vi "RES.vi"(7 "simulazione":bool, 8 "error in (no error)":errorcluster, 11 "Queue Name":string="RES_Q") -> (0 "error out":errorcluster)   [LabVIEW 2019]
uses:
  TypeDef/DEVICE NAME.ctl
  <vilib>/Utility/file.llb/Read Delimited Spreadsheet (string).vi
  Global_All_Data.vi
  Stop lettura res.vi
panel:
  out "Numeric":i32
  in  "Misura Resistomat":bool
  out "T max misura":i32
  out "Precisione mis":dbl
  out "N meas stab":i32
  out "T wait start (s)":i32
  in  "Mode sing?":bool
  out "Reset Device (Don't Reset)":bool
  out "Group Address (0)":i32
  out "Time-out (1.0)":dbl
  out "Baud Rate (9600)":i32
  out "n meas":string
  out "errore resistomat":bool
  out "SCALA":u16
  out "COM-Port (0)":i32
  out "Iteration":i32
  in  "RANGE":u16(ring) items=["20 mOhm", "200 mOhm", "2 Ohm", "20 Ohm", "200 Ohm", "2 kOhm", "20 kOhm", "200 kOhm"]
  in  "CONFIGURE":bool
  in  "stop":bool
  in  "MEASURE":bool
  out "Measuring Value":dbl format="%#_6f OHM"
  out "Communication settings":T1={"COM-Port (0)"=0, "Baud Rate (9600)"=9600, "Time-out (1.0)"=1.0, "Group Address (0)"=0, "Reset Device (Don't Reset)"=FALSE} {"Baud Rate (9600)" items=["1200"=1200, "2400"=2400, "4800"=4800, "9600"=9600, "19200"=19200, "38400"=38400, "56000"=56000, "57600"=57600]; "COM-Port (0)" min=1 max=32 step=1}
  out "N° in queue":i32
  out "variant":variant
  out "STATO":string
  out "LOOP TIME (ms)":u32
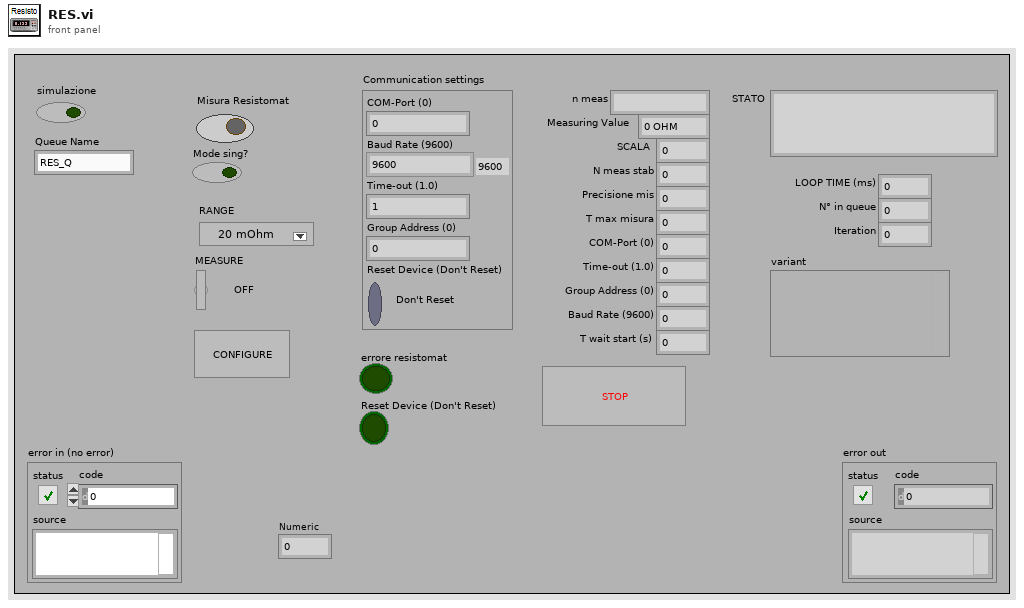
[diagram p1: front panel]
types:
  T1 = cluster{"COM-Port (0)":i32, "Baud Rate (9600)":i32, "Time-out (1.0)":dbl, "Group Address (0)":i32, "Reset Device (Don't Reset)":bool}
  T2 = typedef "DEVICE NAME.ctl" = enum16{"WATTMETRO", "APLUS", "PLC BANCO 1", "PLC RACK", "PLC BANCO 2", "PS", "NI cDAQ", "RESISTOMAT"}
  T3 = typedef "Cluster MISURE.ctl" = cluster{"MISURE NM":T4, "MISURE ALL":T5}
  T4 = typedef "MISURE NM.ctl" = cluster{"Banco":string, "Anno":string, "Numero":string, "Ntabella":string, "Misura":string, "Tipo Prova":string, "ProgressivoAcq":string, "Descrizione":string, "Data_ora":string, "t. acq [h:m:s]":string, "t. acq [min]":string, "t. acq [s]":string, "n [rpm]":string, "f [Hz]":string, "U1[V]":string, "U2 [V]":string, "U3 [V]":string, "U123_media [V]":string, "I1[A]":string, "I2[A]":string, "I3[A]":string, "I123_media [A]*I":string, "I_123_sbil [%]":string, "Ulin[V]":string, "Uc [V]":string, "Uaux [V]":string, "Ilin[A]*I":string, "Imar[A]":string, "Iaux[A]":string, "Uarm[V]":string, "Uecc[V]":string, "Iarm[A]*I":string, "Iecc[A]":string, "pf":string, "P1 [W]":string, "P1 [kW]":string, "Q [VAR]":string, "Q [kVAR]":string, "S [VA]":string, "S [kVA]":string, "P1arm[W]":string, "P1ecc[W]":string, "Parm[kW]":string, "P1ecc[kW]":string, "Cond[uF]":string, "P1_linea_6fili[W]":string, "P1_linea_6fili[kW]":string, "eta_gr_6fili [%]":string, "eta_inverter_6fili [%]":string, "pf_linea_6fili":string, "U4 [V]":string, "U5 [V]":string, "U6 [V]":string, "U456_media [V]":string, "I4 [A]":string, "I5 [A]":string, "I6 [A]":string, "I456_media [A]":string, "C [Nm]*C":string, "Cric [Nm]":string, "Cric\\Cnom":string, "Iric[A]":string, "Iric\\Inom":string, "P2_mecc [W]":string, "P2_mecc [kW]":string, "eta motore [%]":string, "Scorr[%]":string, "Tamb[°C]":string, "R1[ohm]":string, "R2[ohm]":string, "R3[ohm]":string, "Rmedia[ohm]":string, "DT_R1[°C]":string, "DT_R2[°C]":string, "DT_R3[°C]":string, "DT_media[°C]":string, "R_marcia[ohm]":string, "R_aux[ohm]":string, "DT_marcia[°C]":string, "DT_aux[°C]":string, "R_Arm[ohm]":string, "R_Ecc[ohm]":string, "DT_Arm[°C]":string, "DT_Ecc[°C]":string, "TambFreddo[°C]":string, "R1_freddo[ohm]":string, "R2_freddo[ohm]":string, "R3_freddo[ohm]":string, "Rmedia_freddo[ohm]":string, "R_Marcia_freddo[ohm]":string, "R_Aux_freddo[ohm]":string, "R_Arm_freddo[ohm]":string, "R_Ecc_freddo[ohm]":string, "TC1 [°C]":string, "TC2 [°C]":string, "TC3 [°C]":string, "TC4 [°C]":string, "TC5 [°C]":string, "TC6 [°C]":string, "TC7 [°C]":string, "TC8 [°C]":string, "PT1000_1[°C]":string, "PT1000_2[°C]":string, "PT1000_3[°C]":string, "Vdc eccitatrice[V]":string, "Idc eccitatrice[A]":string, "Vdc rotore[V]":string, "Idc rotore[A]":string, "Vac rotore[V]":string, "Iac rotore[V]":string, "V dinamo[V]":string, "Portata Q":string, "Pressione H":string, "U1'[V]":string, "U2'[V]":string, "U3'[V]":string, "I1'[A]":string, "I2'[A]":string, "I3'[A]":string, "U''R-N":string, "U''S-N":string, "U'' T-N":string, "U''R-S":string, "U''R-T":string, "U''S-T":string, "I1''[A]":string, "I2''[A]":string, "I3''[A]":string, "F''[Hz]":string, "P''[kW]":string, "CosFi''":string, "PT1000_4[°C]":string, "Scorta 3":string}
  T5 = typedef "Cluster misure ALL.ctl" = cluster{"Cluster READ NI":T6, "MISURE WT":T9, "Resistenze Resistomat":T10, "INTERFACCIA":T11, "FREDDO resistomat":cluster{"Res Ch1":dbl, "Res Ch2":dbl, "tAMB":dbl, "Res Ch3":dbl}, "STATO PLC 1":T16, "Res Ch2":dbl, "Res Ch2 2":dbl, "FREDDO res meter":cluster{"Res Ch1":dbl, "Res Ch2":dbl, "tAMB":dbl, "Res Ch3":dbl}, "Resistenze Res Meter":T10, "READ SINUS PENTA":T20, "STATO PLC 2":T21, "STATO PLC 3":T25, "DCREG":T29}
  T6 = typedef "Cluster NI.ctl" = cluster{"AI (0-10V)":cluster{"AI 0":dbl, "AI 1":dbl, "AI 2":dbl, "AI 3":dbl, "AI 4":dbl, "AI 5":dbl, "AI 6":dbl, "AI 7":dbl, "AI 8":dbl, "AI 9":dbl, "AI 10":dbl, "AI 11":dbl, "AI 12":dbl, "AI 13":dbl, "AI 14":dbl, "AI 15":dbl, "AI 16":dbl, "AI 17":dbl, "AI 18":dbl, "AI 19":dbl, "AI 20":dbl, "AI 21":dbl, "AI 22":dbl, "AI 23":dbl, "AI 24":dbl, "AI 25":dbl, "AI 26":dbl, "AI 27":dbl, "AI 28":dbl, "AI 29":dbl, "AI 30":dbl, "AI 31":dbl}, "StatoAO_Cdaq[0-10V]":cluster{"AO 1":dbl, "AO 2":dbl, "AO 3":dbl, "AO 4":dbl}, "Contatori [rpm]":cluster{"RPM 1":dbl, "RPM 2":dbl}, "StatoAO_Cdaq [4-20mA]":T7, "StatoDO_Cdaq":T8, "DI":cluster{"Scorta 0":bool, "Scorta 1":bool, "Scorta 2":bool, "Scorta 3":bool, "Scorta 4":bool, "Scorta 5":bool, "Scorta 6":bool, "Scorta 7":bool, "Scorta 8":bool, "Scorta 9":bool, "Scorta 10":bool, "Scorta 11":bool, "Scorta 12":bool, "Scorta 13":bool, "Scorta 14":bool, "Scorta 15":bool, "Scorta 16":bool, "Scorta 17":bool, "Scorta 18":bool, "Scorta 19":bool, "Scorta 20":bool, "Scorta 21":bool, "Scorta 22":bool, "Scorta 23":bool, "Scorta 24":bool, "Scorta 25":bool, "Scorta 26":bool, "Scorta 27":bool, "Scorta 28":bool, "Scorta 29":bool, "Scorta 30":bool, "Scorta 31":bool}, "AI (4-20mA)":cluster{"AI 0":dbl, "AI 1":dbl, "AI 2":dbl, "AI 3":dbl, "AI 4":dbl, "AI 5":dbl, "AI 6":dbl, "AI 7":dbl, "AI 8":dbl, "AI 9":dbl, "AI 10":dbl, "AI 11":dbl, "AI 12":dbl, "AI 13":dbl, "AI 14":dbl, "AI 15":dbl}, "TC [°C]":cluster{"tc 1":dbl, "tc 2":dbl, "tc 3":dbl, "tc 4":dbl}, "NI Read Values":cluster{"RPM":dbl, "Frequency":dbl, "Mod 1":cluster{"Torsiometro 1":dbl, "Torsiometro 2":dbl, "Strin Gauge 1":dbl, "Strin Gauge 2":dbl}, "Mod 2":cluster{"Termocoppia 1":dbl, "Termocoppia 2":dbl, "Termocoppia 3":dbl, "Termocoppia 4":dbl}, "Mod 3":cluster{"PT 100 1":dbl, "PT 100 2":dbl, "PT 100 3":dbl, "PT 100 4":dbl}}}
  T7 = typedef "StatoAO_cdaq.ctl" = cluster{"Cdaq_AO [0-10V] 0 for Torque":dbl, "Cdaq_AO [0-10V] 1":dbl, "Cdaq_AO [0-10V] 2":dbl, "Cdaq_AO [0-10V] 3":dbl}
  T8 = typedef "statoDO_Cdaq.ctl" = cluster{"Scorta 0":bool, "Scorta 1":bool, "Scorta 2":bool, "Scorta 3":bool, "Scorta 4":bool, "Scorta 5":bool, "Scorta 6":bool, "Scorta 7":bool, "Scorta 8":bool, "Scorta 9":bool, "Scorta 10":bool, "Scorta 11":bool, "Scorta 12":bool, "Scorta 13":bool, "Scorta 14":bool, "Scorta 15":bool, "Scorta 16":bool, "Scorta 17":bool, "Scorta 18":bool, "Scorta 19":bool, "Scorta 20":bool, "Scorta 21":bool, "Scorta 22":bool, "Scorta 23":bool, "Scorta 24":bool, "Scorta 25":bool, "Scorta 26":bool, "Scorta 27":bool, "Scorta 28":bool, "Scorta 29":bool, "Scorta 30":bool, "Scorta 31":bool}
  T9 = typedef "MISURE WT.ctl" = cluster{"URMS 1":dbl, "IRMS 1":dbl, "P 1":dbl, "S 1":dbl, "Q 1":dbl, "LAMBDA 1":dbl, "PHI 1":dbl, "F U 1":dbl, "F I 1":dbl, "NONE 1":dbl, "URMS 2":dbl, "IRMS 2":dbl, "P 2":dbl, "S 2":dbl, "Q 2":dbl, "LAMBDA 2":dbl, "PHI 2":dbl, "F U 2":dbl, "F I 2":dbl, "NONE 2":dbl, "URMS 3":dbl, "IRMS 3":dbl, "P 3":dbl, "S 3":dbl, "Q 3":dbl, "LAMBDA 3":dbl, "PHI 3":dbl, "F U 3":dbl, "F I 3":dbl, "NONE 3":dbl, "URMS SIGMA":dbl, "IRMS SIGMA":dbl, "P SIGMA":dbl, "S SIGMA":dbl, "Q SIGMA":dbl, "LAMBDA SIGMA":dbl, "PHI SIGMA":dbl, "F U SIGMA":dbl, "F I SIGMA":dbl, "NONE 4":dbl}
  T10 = typedef "ClusterRes.ctl" = cluster{"Res Ch1":dbl, "Res Ch2":dbl, "Res Ch3":dbl, "Tamb":dbl}
  T11 = typedef "INTERFACCIA.ctl" = cluster{"AI":cluster{"Portate":T12[], "Pressioni":T12[], "Coppie[Nm]":T12[], "Valvole prop %":T12[], "RPM":T12[], "Livelli":T12[], "Temperature":T12[], "Riferimenti %":T12[], "TENSIONI":T12[], "CORRENTI":T12[]}, "DI (logici)":cluster{"Start da pulsantiera":bool, "Stop da pulsantiera":bool, "Reset da pulsantiera":bool, "Sistema OK":bool, "Collaudo abilitato":bool, "Potenza trifase abilitata":bool, "Potenza monofase abilitata":bool, "Potenza DC abilitata":bool, "Potenza DC ECC abilitata":bool, "Start alimentazione AC":bool, "Start alimentazione DC":bool, "Start DC eccitazione":bool, "Teleruttore WT abilitato":bool, "Teleruttore Resistomat abilitato":bool, "Teleruttore corto fasi":bool, "Ramo 1 resistomat":bool, "Ramo 2 resistomat":bool, "Ramo 3 resistomat":bool, "B1 Scelta linea elettrica 1":bool, "B1 Scelta linea elettrica 2":bool, "B1 Scelta linea elettrica 3":bool, "B1 Scelta linea elettrica 4":bool, "B1 Scelta linea elettrica 5":bool, "B2 Scelta linea elettrica 1":bool, "B2 Scelta linea elettrica 2":bool, "B2 Scelta linea elettrica 3":bool, "B2 Scelta linea elettrica 4":bool, "B2 Scelta linea elettrica 5":bool, "Rotore bloccato 1":bool, "Rotore bloccato 2":bool, "FRENO 1 abilitato":bool, "FRENO 1 run":bool, "FRENO 1 senso rotaz":bool, "FRENO 1 ctrl velocità":bool, "FRENO 2 abilitato":bool, "FRENO 2 run":bool, "FRENO 2 senso rotaz":bool, "FRENO 2 ctrl velocità":bool, "ALIM 1 abilitato":bool, "ALIM 1 run":bool, "ALIM 2 abilitato":bool, "ALIM 2 run":bool, "ALIM 3 abilitato":bool, "ALIM 3 run":bool, "FRENO 1 ctrl coppia":bool, "FRENO 2 ctrl coppia":bool, "FRENO 3 ctrl coppia":bool, "DI (logici) aggiuntivi impianto":cluster{"Solo freno abilitato":bool, "Carico resistivo abilitato":bool, "AFE+freno abilitato":bool, "Protezioni chiuse":bool, "Start potenza AFE":bool, "AFE in marcia":bool}, "Misura corrente diretta WT":bool, "Misura corrente sens ext":bool, "Sens ext abilitati":bool}, "AO non scalati":T14, "AO scalati":T14, "DO (logici)":T15}
  T12 = typedef "ClusterMisura_e_Unità_INPUT.ctl" = cluster{"Misura":dbl, "UM":T13, "Descrizione":string}
  T13 = typedef "UnitàMisura.ctl" = enum16{"V", "mA", "Bar", "RPM", "m3/s", "m3/min", "m3/h", "l/s", "l/min", "in3/min", "ft3/min", "gpm", "igpm", "igph", "%", "°C", "m", "Nm", "A"}
  T14 = typedef "Lista AO sistema.ctl" = cluster{"FRENO1 rif vel":dbl, "FRENO1 rif Coppia":dbl, "FRENO2 rif vel":dbl, "FRENO2 rif Coppia":dbl, "ALIM1 rif V":dbl, "ALIM1 rif F":dbl, "ALIM2 rif V":dbl, "ALIM2 rif F":dbl, "ALIM3 rif V":dbl, "ALIM3 rif F":dbl, "Fnom keb":dbl, "Rpm nom keb":dbl, "Pnom keb":dbl, "Inom keb":dbl, "Vnom keb":dbl, "Rpm max keb":dbl, "Tempo rampa keb":dbl, "Tipo Mot keb":dbl, "FRENO  rif Coppia ":dbl, "FRENO  rif  Corrente":dbl}
  T15 = typedef "DOinterfaccia.ctl" = cluster{"Scelta banco 1":bool, "Scelta banco 2":bool, "Scelta banco 3":bool, "FRENO 1 abilita":bool, "FRENO 1 start":bool, "FRENO 1 senso rotaz":bool, "FRENO 1 ctrl velocità":bool, "FRENO 2 abilita":bool, "FRENO 2 start":bool, "FRENO 2 senso rotaz":bool, "FRENO 2 ctrl velocità":bool, "ALIM 1 abilita":bool, "ALIM 1 start":bool, "ALIM 2 abilita":bool, "ALIM 2 start":bool, "ALIM 3 abilita":bool, "ALIM 3 start":bool, "Abilita linea trifase":bool, "Abilita linea monofase":bool, "Abilita linea dc":bool, "Abilita linea dc eccit":bool, "B1 Linea elettrica 1":bool, "B1 Linea elettrica 2":bool, "B1 Linea elettrica 3":bool, "B1 Linea elettrica 4":bool, "B1 Linea elettrica 5":bool, "B2 Linea elettrica 1":bool, "B2 Linea elettrica 2":bool, "B2 Linea elettrica 3":bool, "B2 Linea elettrica 4":bool, "B2 Linea elettrica 5":bool, "Start potenza AC":bool, "Stop pontenza AC":bool, "Start potenza DC":bool, "Stop potenza DC":bool, "Start potenza eccitaz":bool, "Stop potenza eccitaz":bool, "Reset allarmi":bool, "watchdog":bool, "Scala torsiometro B1":bool, "Controllo torsiom B1":bool, "Scala torsiometro B2":bool, "Controllo torsiom B2":bool, "Teleruttore WT abilita":bool, "Teleruttore Resistomat abilita":bool, "Teleruttore corto fasi":bool, "Ramo 1 resistomat":bool, "Ramo 2 resistomat":bool, "Ramo 3 resistomat":bool, "Collaudo in corso":bool, "Allarme presente":bool, "Enable Res Meter":bool, "Bypass Res Meter":bool, "2nd canale Res Meter":bool, "Scala 200/2000 res meter":bool, "Taratura res meter":bool, "FRENO 1 ctrl coppia":bool, "FRENO 2 ctrl coppia":bool, "FRENO 3 ctrl coppia":bool, "Aggiuntivi impianto":cluster{"Senso rotazione alim 1":bool, "Senso rotazione alim 2":bool}, "ALIM 1 stop":bool, "ALIM 2 stop":bool, "ALIM 3 stop":bool, "FRENO 1 stop":bool, "FRENO 2 stop":bool, "FRENO 3 stop":bool, "B1 configurazione freno B":bool, "B2 configurazione freno B":bool, "Abilita scrittura KEB":bool, "Bench Selection (0-B1,1-B2)":bool, "Select current mode":bool, "Select torque mode":bool, "Select speed mode":bool, "Start":bool, "Stop":bool, "Block":bool, "Enable Force mode":bool, "Abilita linea 125 A":bool, "Abilita linea 63 A":bool, "Abilita linea 16 A":bool, "Aum Tensione Variac":bool, "Dim Tesnione Variac":bool, "Abilita ellectro stractura":bool, "Risprinito Emergence":bool, "Abilita collaudo":bool, "Disabilita collaudo":bool, "External Alaram":bool, "Enable external program":bool, "Reset":bool, "Abilita Ingresso Variac":bool, "Abilita Ventilatore Variac":bool, "Abilita Uscita Variac ":bool}
  T16 = typedef "STATO PLC 1.ctl" = cluster{"USCITE PLC":T17, "Stato DI_PLC":cluster{"Sistema OK":bool, "Rotore bloccato":bool, "Scorta 1":bool, "Prova diretto inverter":bool, "Prova con filtro LC":bool, "Teleruttore WT abilitato":bool, "Alim sinus penta abilitato":bool, "Alim sinus penta in marcia":bool, "Freno abilitato":bool, "Freno in marcia":bool, "Senso rotazione freno":bool, "Potenza abilitata":bool, "Scorta 3":bool, "Scorta 4":bool, "scorta 5":bool, "scorta 6":bool}, "AI plc":cluster{"Allarmi 1":dbl, "Allarmi 2":dbl, "Scorta 1":dbl, "Scorta 2":dbl, "RPM mot prova":dbl, "I mot prova":dbl, "RPM freno":dbl, "I freno":dbl, "Scorta 3":dbl, "Scorta 4":dbl}}
  T17 = typedef "Uscite PLC 1.ctl" = cluster{"AO (real) 2":cluster{"SCORTA 1":dbl, "SCORTA 2":dbl, "SCORTA 3":dbl, "SCORTA 4":dbl, "SCORTA 5":dbl, "SCORTA 6":dbl, "SCORTA 7":dbl, "SCORTA 8":dbl}, "statoAO_PLC out":T18, "DO (bit)":T19}
  T18 = typedef "statoAO_plc_1.ctl" = cluster{"Rif Lim coppia freno [%]":dbl, "Rif rpm freno [%]":dbl, "Rif coppia freno [%]":dbl, "Rif V alimentatore [%]":dbl, "Rif F alimentatore [%]":dbl}
  T19 = typedef "StatoDO_PLC_1.ctl" = cluster{"Scelta banco 1":bool, "Set dati motore freno 2":bool, "Diretto inverter":bool, "Filtro LC":bool, "Marcia ALIM (1s)":bool, "Marcia FRENO (1s)":bool, "Stop AFE (1s)":bool, "Stop freno (1s)":bool, "Reset allarmi":bool, "Watchdog":bool, "Senso rotazione":bool, "Abilita collaudo (1s)":bool, "Disabilita collaudo (1s)":bool, "Abilitazione ALIM":bool, "Abilitazione FRENO":bool, "Teleruttore WT":bool, "Senso rot motore prova":bool, "Scorta 7":bool, "Scorta 8":bool, "Scorta 9":bool, "Scorta 10":bool, "Scorta 11":bool, "Scorta 12":bool, "Scorta 13":bool}
  T20 = typedef "Parametri inverter letti.ctl" = cluster{"Menù Misure motore (M000-M030)":cluster{"Rif vel a regime (int)":u16, "Rif vel a regime (dec)":u16, "Rif vel dopo rampe (int)":u16, "Rif vel dopo rampe (dec)":u16, "RPM motore (int)":u16, "RPM motore (dec)":u16, "FREQout inverter":u16, "Rif coppia a regime(Nm)":u16, "Richiesta di coppia (Nm)":u16, "Coppia generata dal motore(Nm)":u16, "Rif coppia a regime(%)":u16, "Richiesta di coppia (%)":u16, "Coppia generata dal motore(%)":u16, "Coppia max richiesta prima delle rampe(Nm)":u16, "Coppia max richiesta dopo le rampe(Nm)":u16, "Limite di velocità prima delle rampe":u16, "Limite di velocità dopo le rampe":u16, "Coppia max richiesta prima delle rampe(%)":u16, "Coppia max richiesta dopo le rampe(%)":u16, "Rif di flusso":u16, "Corrente di uscita":u16, "Capacità termica del motore":u16, "Tensione di uscita":u16, "Potenza di uscita":u16, "Energia consumata (LSword)":u16, "Energia consumata (MSword)":u16, "Tensione bus DC":u16, "Tensione di rete":u16}, "Menù regolatore PID (M018-M024)":cluster{"Rif PID a regime(%)":u16, "Rif pid dopo rampe(%)":u16, "Retroazione del pid(%)":u16, "Errore del pid(%)":u16, "uscita del pid(%)":u16, "Rif del pid dopo le rampe":u16, "Retroazione del pid":u16}, "Menù ingressi digitali (M031-M036)":cluster{"Ingressi digitali ritardati":u16, "Ingressi digitali istantanei":u16, "Moresettiera comando loc":u16, "Morsett comando da seriale":u16, "Morsett comando bus di campo":u16, "Ing dig ausiliari da morsettiera":u16, "Ing dig ausiliari da seriale":u16}, "Menù riferimenti (M037-M051)":cluster{"Rif analog est REF":u16, "Rif analog est AIN1":u16, "Rif analog est AIN2":u16, "Rif analog est XAIN4":u16, "Rif analog est XAIN5":u16, "Rif velocità da seriale(int)":u16, "Rif velocità bus di campo(int)":u16, "Rif coppia da seriale":u16, "Rif coppia bus di campo":u16, "Rif del PID da seriale":u16, "Rif del PID da bus di campo":u16, "Retroazione del PID da seriale":u16, "Retroazione del PIDda bus di campo":u16, "Rif da encoder":u16, "Rif in frequenza":u16, "Rif velocità da seriale(dec)":u16, "Rif velocità bus di campo(dec)":u16}, "Menù rampe (P009-P033)":cluster{"Tempo di dec rampa di vel 1":u16, "Tempo di acc rampa di vel 2":u16, "Tempo di dec rampa di vel 2":u16, "Tempo di acc rampa di vel 1":u16, "Unità di mis tempi rampe vel 1/2":u16, "Tempo di acc rampa di vel 3":u16, "Tempo di dec rampa di vel 3":u16, "Tempo di acc rampa di vel 4":u16, "Tempo di dec rampa di vel 4":u16, "Unità di mis tempi rampe vel 3/4":u16, "Selettore arrottondam rampe":u16, "Tempo di arrotond iniz rampa acc":u16, "Tempo di arrotond finale rampa acc":u16, "Tempo di arrotond iniz rampa dec":u16, "Tempo di rampa di salita rif coppia":u16, "Tempo di rampa di discesa rif coppia":u16, "Unità di misura rampa coppia":u16, "Tempo rampa acc marcia jog":u16, "Tempo rampa dec marcia jog":u16, "Reset acc ai cambi pendenza":u16, "rampa di acc in fire mode":u16, "rampa di dec in fire mode":u16, "Tempo di arrotond finale rampa dec":u16}, "Menù controllo motore(C008-C128)":cluster{"Numero motori configurati":u16, "Tipo algoritmo di controllo Mot1":u16, "Tipo rif Mot1":u16, "Tensione nominale rete":u16, "Retroaz di vel da encoder Mot1":u16, "Tipo curva V/f Mot1":u16, "Rotazione delle fasi Mot1":u16, "Freq nominale del motore Mot1":u16, "RPM nominali del motore Mot1":u16, "Potenza nominale del motore Mot1":u16, "Corrente nominale del motore Mot1":u16, "Tensione nominale del motore mot1":u16, "Potenza a vuoto del motore Mot1":u16, "Corrente a vuoto del motore Mot1":u16, "Resistenza statorica del motore Mot1":u16, "Induttanza di dispersione Mot1":u16, "Induttanza mutua motore":u16, "Costante di tempo rotorica":u16, "Costante di tempo filtro pb":u16, "Velocità minima motore":u16, "Velocità massima motore":u16}, "Menù configurazione PID":cluster{"Selezione riferimento n.1":u16, "Selezione retroazione n.1":u16, "Modalità di fuzionamento PID":u16, "Termine derivativo calcolato su err o mis":u16, "Proporz moltiplica deriv e integrale":u16, "Azione del PID":u16}, "ID":dbl, "Menù uscite digitali":cluster{"MDO4 Inverter pronto":u16}, "Fcarrier":cluster{"Fcarrier Min (Hz)":u16, "Fcarrier Max (Hz)":u16}, "stato inverter M089":dbl, "Riferimenti":cluster{"Rif tensione":u16, "Rif velocità":u16}, "Comunicazione":bool, "Modalità stop":dbl}
  T21 = typedef "STATO PLC 2.ctl" = cluster{"USCITE PLC":T22, "Stato DI_PLC":cluster{"Sistema ok":bool, "Relè Resistomat abilitato":bool, "Freno abilitato":bool, "Freno in marcia":bool, "scorta b":bool, "scorta a":bool, "scorta 1":bool, "scorta 2":bool, "scorta 3":bool, "scorta 4":bool, "Scorta 5":bool, "Scorta 6":bool, "Scorta 7":bool, "Scorta 8":bool, "Scorta 9":bool, "Scorta 10":bool}, "AI plc":cluster{"Allarmi 1":dbl, "Allarmi 2":dbl, "TC 1":dbl, "TC 2":dbl, "TC 3":dbl, "TC 4":dbl, "TC 5":dbl, "TC 6":dbl, "TC 7":dbl, "TC 8":dbl, "PT1000 1":dbl, "PT1000 2":dbl, "PT1000 3":dbl, "PT1000 4":dbl}}
  T22 = typedef "Uscite PLC 2.ctl" = cluster{"AO (real) 2":cluster{"SCORTA 1":dbl, "SCORTA 2":dbl, "SCORTA 3":dbl, "SCORTA 4":dbl, "SCORTA 5":dbl, "SCORTA 6":dbl, "SCORTA 7":dbl, "SCORTA 8":dbl}, "statoAO_PLC out":T23, "DO (bit)":T24}
  T23 = typedef "statoAO_plc_2.ctl" = cluster{"Condensatori":dbl, "Scorta 1":dbl, "Scorta 2":dbl}
  T24 = typedef "StatoDO_PLC_2.ctl" = cluster{"Relè misura resistomat":bool, "Misura res ramo 1":bool, "Misura res ramo 2":bool, "Misura res ramo 3":bool, "Scelta banco 2":bool, "Scala Torsiometro":bool, "Ctrl torsiometro":bool, "Select current mode":bool, "Select Torque mode":bool, "Select speed mode":bool, "Watchdog":bool, "Scorta":bool, "Scorta 2":bool, "Scorta 3":bool, "Scorta 4":bool, "Scorta 5":bool, "Bench selection":bool, "External alarm":bool, "Enable external program":bool, "Reset allarmi":bool, "Start":bool, "Stop":bool, "Block":bool, "Scorta 6":bool}
  T25 = typedef "STATO PLC 3.ctl" = cluster{"USCITE PLC":T26, "Stato DI_PLC":cluster{"Sistema OK":bool, "Rotore bloccato":bool, "Filtro LC":bool, "Bypass Filtro LC":bool, "Scelta Trasformatore":bool, "Scelta Bypass trasformatore":bool, "Teleruttore wt abilitato":bool, "Alimentatore abilitato":bool, "Alimentatore in marcia":bool, "Scorta 1":bool, "Scorta 2":bool, "Scorta 3":bool, "Potenza abilitata":bool, "Alimentatore in allarme":bool, "Scorta 4":bool, "Conferma dati KEB":bool, "Scorta 5":bool, "Warning Inverter Alimentatore":bool, "Variac Abilitato":bool, "Linea 125 A abilitata":bool, "Linea 63 A abilitata":bool, "Linea 16 A abilitata":bool, "Scorta 6":bool, "Enable force mode":bool}, "AI plc":cluster{"Allarmi 1":dbl, "Allarmi 2":dbl, "RPM motore prova":dbl, "Corrente motore prova":dbl, "RPM freno":dbl, "Corrente freno":dbl, "Tipo motore keb":dbl, "I nom keb":dbl, "RPM nom keb":dbl, "V nom keb":dbl, "F nom keb":dbl, "T rampa keb":dbl, "scorta":dbl, "Scorta 2":dbl}}
  T26 = typedef "Uscite PLC 3.ctl" = cluster{"AO (real) 2":cluster{"SCORTA 1":dbl, "SCORTA 2":dbl, "SCORTA 3":dbl, "SCORTA 4":dbl, "SCORTA 5":dbl, "SCORTA 6":dbl, "SCORTA 7":dbl, "SCORTA 8":dbl}, "statoAO_PLC out":T27, "DO (bit)":T28}
  T27 = typedef "statoAO_plc_3.ctl" = cluster{"Rif velocità alimentatore":dbl, "Scorta":dbl, "Tipo Motore  keb":dbl, "I nom keb":dbl, "RPM nom keb":dbl, "V nom keb":dbl, "F nom keb":dbl, "t rampa keb":dbl}
  T28 = typedef "StatoDO_PLC_3.ctl" = cluster{"Select linea Inverter":bool, "Abilita sense wattmetro":bool, "Bypass filtro LC":bool, "Filtro LC":bool, "Bypass trasformatore":bool, "Trasformatore":bool, "Abilita uscite variac":bool, "Abilita linea 125 A":bool, "Abilita linea 63 A":bool, "Abilita linea 16 A":bool, "Abilita Scrittura Dati Keb":bool, "Abilita alimentatore":bool, "Marcia alimentatore (1s)":bool, "Stop alimentatore (1s)":bool, "Senso rot mot prova":bool, "Watchdog":bool, "Aumenta tensione variac":bool, "Diminuisci tensione variac ":bool, "Blocco elettroserrature":bool, "Ripristino emergence":bool, "Abilita ingresso variac":bool, "Abilita ventilatore variac":bool, "Reset Allarm":bool, "Scorta 1":bool, "Scorta 2":bool, "Scorta 3":bool, "Scorta 4":bool, "Scorta 5":bool, "Scorta 6":bool, "Scorta 7":bool, "Scorta 8":bool, "Scorta 9":bool, "Abilita collaudo":bool, "Disabilita collaudo ":bool, "Scorta 10":bool, "Scorta 11":bool, "Scorta 12":bool, "Scorta 13":bool, "Scorta 14":bool, "Scorta 15":bool}
  T29 = typedef "Parametri DCREG letti.ctl" = cluster{"Parametri di misura":cluster{"M000":dbl, "M001":dbl, "M002":dbl, "M003":dbl, "M004":dbl, "M005":dbl, "M006":dbl, "M007":dbl, "M008":dbl, "M009":dbl, "M010":dbl, "M011":dbl, "M012":dbl, "M013":dbl, "M014":dbl, "M015":dbl, "M016":dbl, "M017":dbl, "M018":dbl, "M019":dbl, "M020":dbl, "M021":dbl, "M022":dbl, "M023":dbl, "M024":dbl, "M025":dbl, "M026":dbl, "M027":dbl, "M028":dbl, "M029":dbl, "M030":dbl, "M031":dbl}, "Parametri di programmazione":cluster{"P000":dbl, "P001":dbl, "P002":dbl, "P003":dbl, "P004":dbl, "P005":dbl, "P006":dbl, "P010":dbl, "P011":dbl, "P012":dbl, "P013":dbl, "P014":dbl, "P015":dbl, "P016":dbl, "P030":dbl, "P031":dbl, "P032":dbl, "P033":dbl, "P034":dbl, "P035":dbl, "P036":dbl, "P037":dbl, "P038":dbl, "P039":dbl, "P040":dbl, "P050":dbl, "P051":dbl, "P052":dbl, "P053":dbl, "P054":dbl, "P055":dbl, "P056":dbl, "P057":dbl, "P058":dbl, "P059":dbl, "P060":dbl, "P061":dbl, "P062":dbl, "P070":dbl, "P071":dbl, "P073":dbl, "P074":dbl, "P076":dbl, "P077":dbl, "P079":dbl, "P080":dbl, "P082":dbl, "P083":dbl, "P084":dbl, "P085":dbl, "P086":dbl, "P087":dbl, "P088":dbl, "P100":dbl, "P101":dbl, "P102":dbl, "P103":dbl, "P104":dbl, "P110":dbl, "P111":dbl, "P120":dbl, "P121":dbl, "P122":dbl, "P123":dbl, "P124":dbl, "P125":dbl, "P126":dbl, "P127":dbl, "P128":dbl, "P129":dbl, "P130":dbl, "P131":dbl, "P132":dbl, "P133":dbl, "P134":dbl, "P150":dbl, "P151":dbl, "P152":dbl, "P153":dbl, "P154":dbl, "P155":dbl, "P156":dbl, "P157":dbl, "P158":dbl, "P170":dbl, "P171":dbl, "P172":dbl, "P173":dbl, "P174":dbl, "P175":dbl, "P176":dbl, "P177":dbl, "P178":dbl, "P179":dbl, "P180":dbl, "P181":dbl, "P182":dbl, "P183":dbl, "P184":dbl, "P185":dbl, "P186":dbl, "P187":dbl, "P188":dbl, "P189":dbl, "P190":dbl, "P191":dbl, "P192":dbl, "P193":dbl, "P194":dbl, "P195":dbl, "P196":dbl, "P197":dbl, "P198":dbl, "P199":dbl, "P211":dbl, "P212":dbl, "P213":dbl, "P214":dbl, "P215":dbl, "P216":dbl, "P217":dbl, "P221":dbl, "P222":dbl, "P223":dbl, "P224":dbl, "P230":dbl, "P231":dbl, "P240":dbl, "P250":dbl, "P251":dbl}, "Parametri di configurazione":cluster{"C000":dbl, "C001":dbl, "C002":dbl, "C010":dbl, "C011":dbl, "C012":dbl, "C014":dbl, "C015":dbl, "C016":dbl, "C017":dbl, "C018":dbl, "C030":dbl, "C050":dbl, "C051":dbl, "C052":dbl, "C060":dbl, "C061":dbl, "C062":dbl, "C063":dbl, "C070":dbl, "C072":dbl, "C074":dbl, "C090":dbl, "C091":dbl, "C092":dbl, "C093":dbl, "C094":dbl, "C100":dbl, "C101":dbl, "C102":dbl, "C103":dbl, "C105":dbl, "C106":dbl, "C107":dbl, "C108":dbl, "C110":dbl, "C111":dbl, "C112":dbl, "C120":dbl, "C121":dbl, "C122":dbl, "C130":dbl, "C131":dbl, "C132":dbl, "C133":dbl, "C134":dbl, "C135":dbl, "C141":dbl, "C142":dbl, "C143":dbl, "C150":dbl, "C151":dbl, "C153":dbl, "C154":dbl, "C155":dbl, "C156":dbl, "C157":dbl, "C158":dbl, "C159":dbl, "C160":dbl, "C161":dbl, "C162":dbl, "C163":dbl, "C164":dbl, "C165":dbl, "C170":dbl}, "Codice allarme":dbl, "Comunicazione":bool}
  T30 = enum32{"Invalid", "Standard", "Closed", "Hidden", "Minimized", "Maximized"}
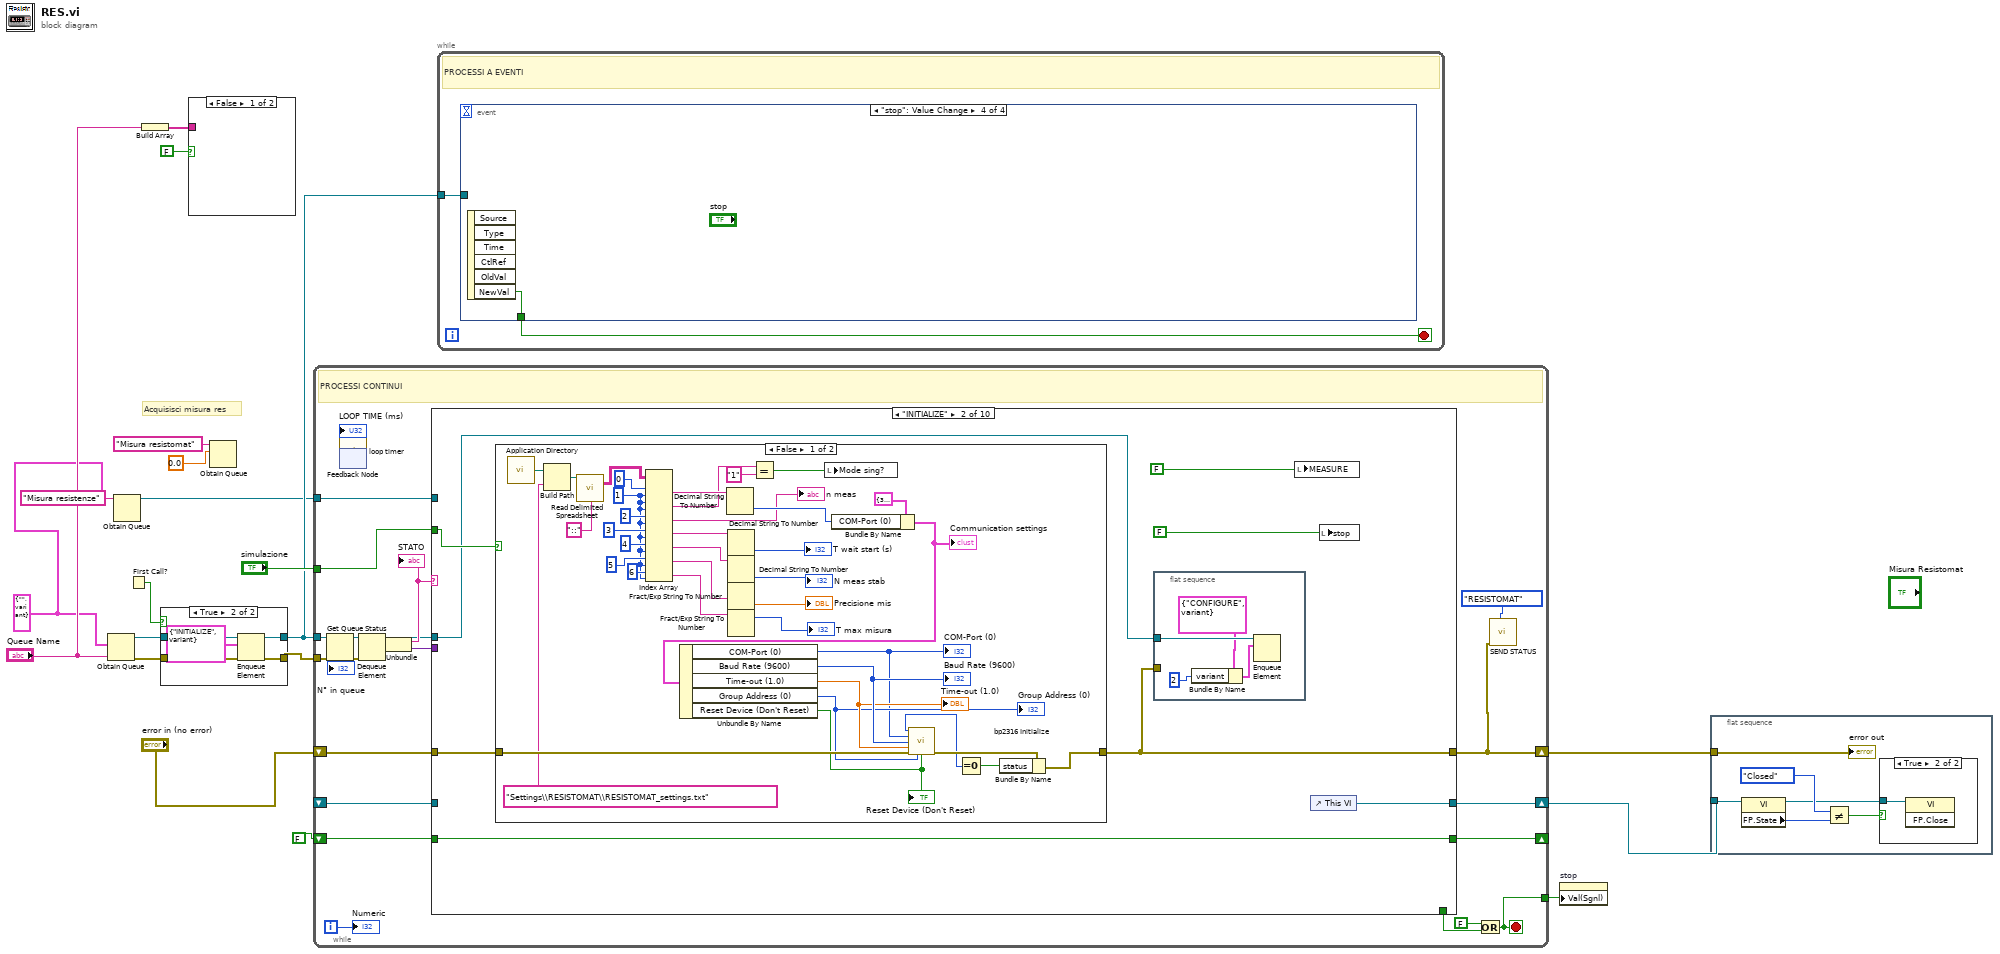
[diagram p0: block diagram]
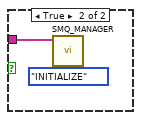
[diagram p3: hidden frame]
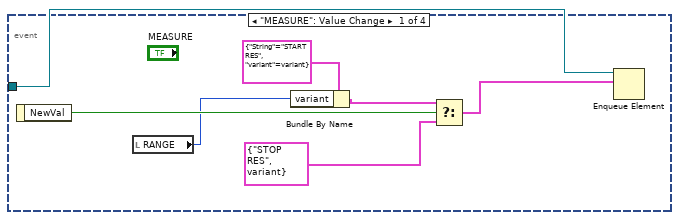
[diagram p4: hidden frame]
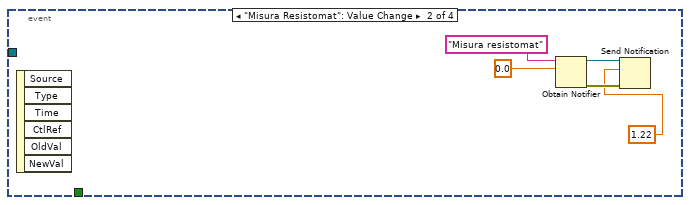
[diagram p5: hidden frame]
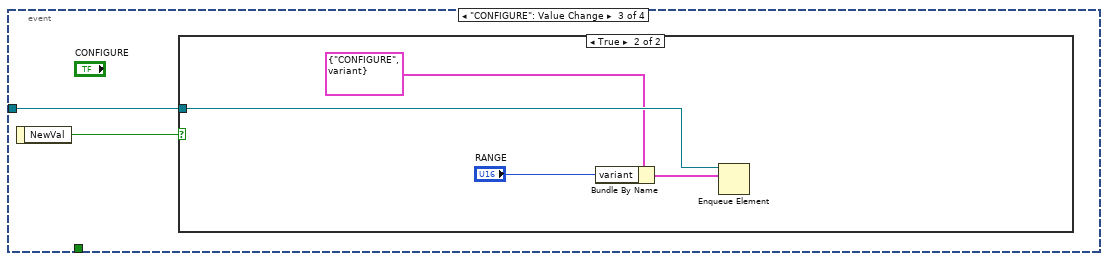
[diagram p6: hidden frame]
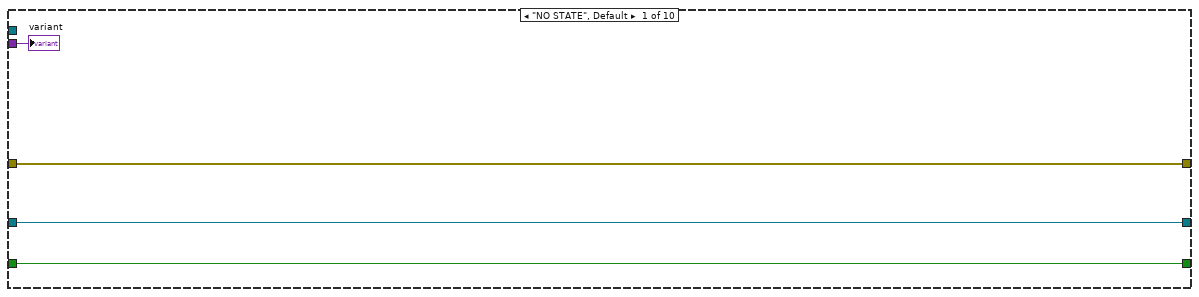
[diagram p9: hidden frame]
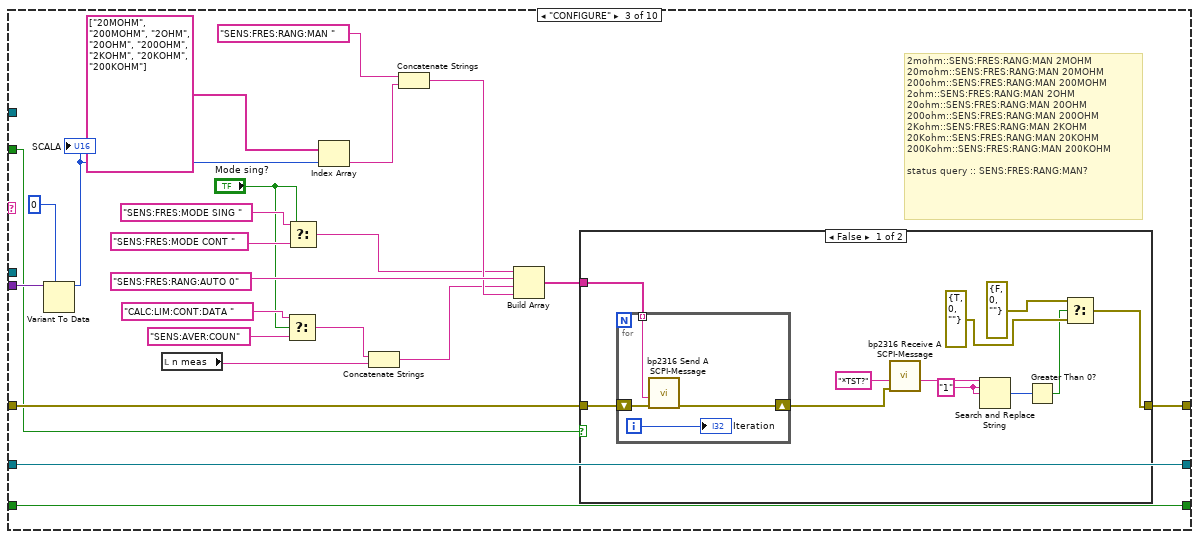
[diagram p11: hidden frame]
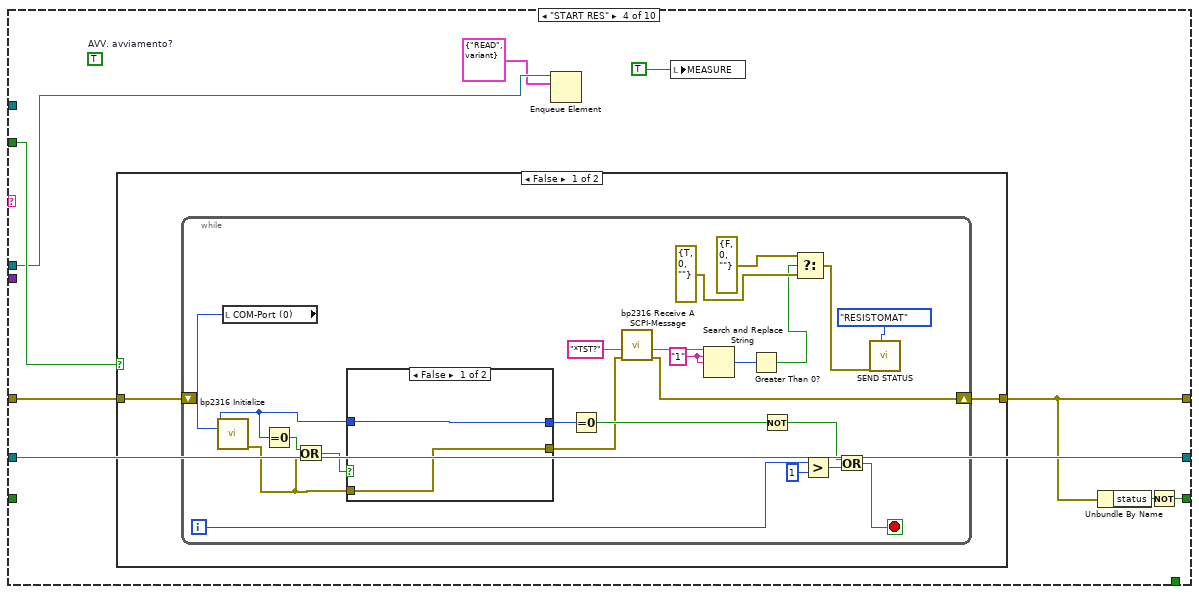
[diagram p13: hidden frame]
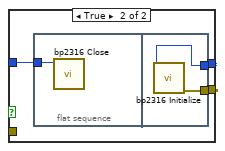
[diagram p14: hidden frame]
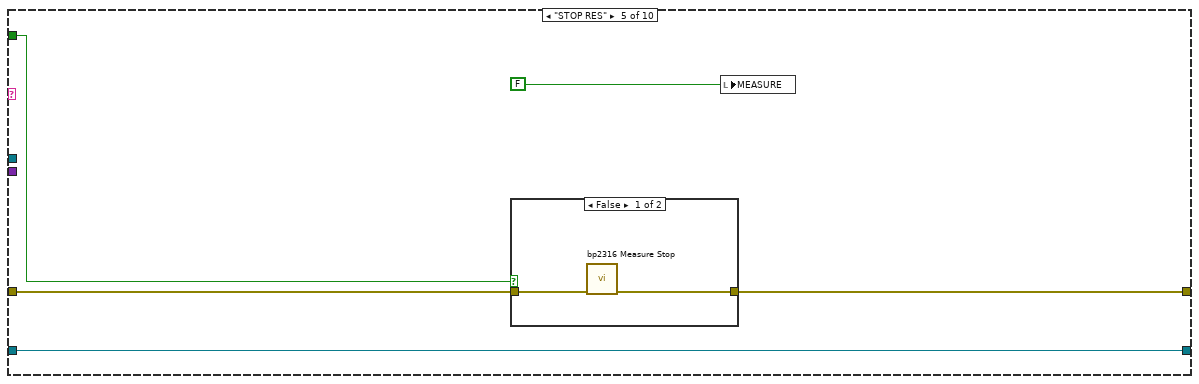
[diagram p16: hidden frame]
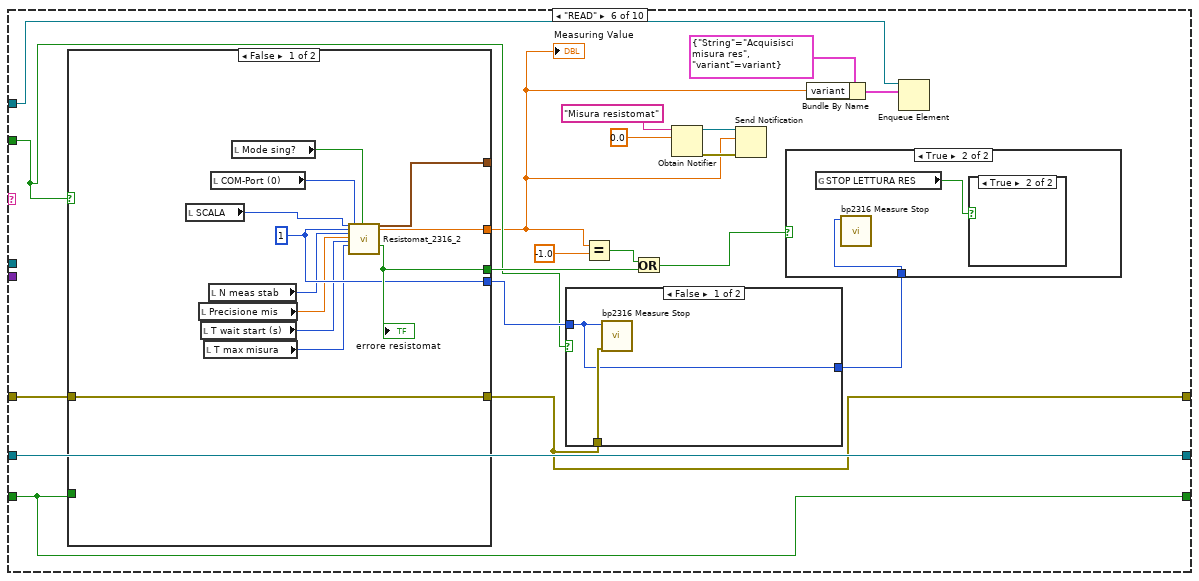
[diagram p18: hidden frame]
diagram:
  w3 = cluster{"String":string, "variant":variant} {"String"="", "variant"=variant} ("element")
  # "Acquisisci misura res"
  n1 = Obtain Queue(name (unnamed)="Queue Name", element data type=w3) -> (queue out=w14:refnum<queue>, error out=w13:errorcluster)  [unwired: 3 in, 1 out]
  n2 = Obtain Queue(name (unnamed)="Misura resistenze", element data type=w3) -> (queue out=w5:refnum<queue>)  [unwired: 3 in, 2 out]
  n3 = First Call?() -> (First Call?: T/F=w8:bool)
  n4 = Build Array("Queue Name") -> (w10:string[])
  n5 = case shown="True" w8 {
    tunnel: w14 -> [w21 w26]
    tunnel: w13 -> [w20 w25]
    tunnel: [w21 w24] -> w7
    tunnel: [w20 w23] -> w12
    frame False {
    }
    frame True {
      n6 = Enqueue Element(queue=w26, element=cluster{"String":string, "variant":variant} {"String"="INITIALIZE", "variant"=variant}, error in (no error)=w25) -> (queue out=w24:refnum<queue>, error out=w23:errorcluster)  [unwired: 1 in, 1 out]
    }
  }
  n7 = case shown="False" FALSE {
    tunnel: w10 -> [_ w27]
    frame False {
    }
    frame True {
      n8 = call <userlib>:"SMQ_MANAGER.vi"("Function"=enum16{"INITIALIZE", "ENQUEUE", "STOP ALL"}."INITIALIZE", "Queue array"=w27) -> ()  [unwired: 9 in, 1 out]
    }
  }
  n9 = Obtain Queue(name (unnamed)="Misura resistomat", element data type=0.0) -> ()  [unwired: 3 in, 3 out]
  n10 = while {
    shift-right: [w52] -> w18
    shift-left: _ -> [w51]
    shift-right: [w30] -> w4
    shift-left: "error in (no error)" -> [w50]
    tunnel: w7 -> [w44]
    tunnel: w12 -> [w43]
    tunnel: "simulazione" -> [w45]
    shift-right: [w37] -> _
    shift-left: FALSE -> [w36]
    tunnel: [w35] -> w15
    tunnel: w5 -> [w32]
    i -> [w29]
    stop <- w35 stop-if-true
    # "PROCESSI CONTINUI"
    n11 = Get Queue Status(queue=w44, error in (no error)=w43) -> (queue out=w41:refnum<queue>, error out=w42:errorcluster, # elements in queue=→"N° in queue":i32)  [unwired: 1 in, 5 out]
    n12 = feedback #1() -> (w38:u32)  [unwired: 1 in]
    n13 = call <userlib>:"loop timer.vi"("millisecond timer IN"=w38) -> ("millisecond timer OUT"=w39:u32, "LOOP TIME (ms)"=→"LOOP TIME (ms)":u32)  [unwired: 9 in]
    n14 = feedback-in #1(w39) -> ()
    n15 = Dequeue Element(queue=w41, error in (no error)=w42) -> (queue out=w34:refnum<queue>, element=w49:cluster{"String":string, "variant":variant})  [unwired: 1 in, 2 out]
    n16 = Unbundle(w49) -> ("String"=w48:string, "variant"=w47:variant)
    "STATO" <- w48
    n17 = case shown="\"INITIALIZE\"" w48 {
      tunnel: [_ _ _ _ _ _ _ _ _ TRUE] -> w46
      tunnel: [w57 w65 w131 w156 w195 w217 w256 w258 w265 w270] -> w52
      tunnel: w51 -> [w57 _ w131 w156 w195 w217 w256 w258 w265 w270]
      tunnel: w50 -> [w56 w63 w129 w148 w194 w216 w255 w259 w263 w268]
      tunnel: [w56 w58 w128 w151 w193 w208 w255 w259 w261 w267] -> w30
      tunnel: w47 -> [w55 _ w124 _ _ _ _ _ _ _]
      tunnel: w45 -> [_ w64 w116 w155 w192 w210 _ _ _ w269]
      tunnel: [w54 w60 w130 w153 _ w215 _ w257 _ _] -> w37
      tunnel: w36 -> [w54 w60 w130 _ _ w215 _ w257 _ _]
      tunnel: w34 -> [_ w59 _ w150 _ _ _ _ w264 _]
      tunnel: w32 -> [_ _ _ _ _ w207 _ _ _ _]
      frame "NO STATE", Default {
        "variant" <- w55
      }
      frame "INITIALIZE" {
        n18 = case shown="False" w64 {
          tunnel: w63 -> [w107 w108]
          tunnel: [w98 w108] -> w58
          frame False {
            w72 = 1 ("disabled index (col)")
            n19 = call <vilib>:"Application Directory.vi"() -> ("Application Directory"=w95:path)
            n20 = Build Path(base path=w95, name or relative path="Settings\\RESISTOMAT\\RESISTOMAT_settings.txt") -> (appended path=w93:path)
            n21 = call-poly <vilib>:"Read Delimited Spreadsheet.vi"("file path (dialog if empty)"=w93, "delimiter (\\t)"="::" ("delimiter (\\t)")) -> ("all rows"=w90:string[][])  [unwired: 8 in, 5 out]
            n22 = Index Array(array=w90, index (row) #1=0 ("disabled index (row)"), index (col) #1=w72, index (row) #2=w72, index (col) #2=w72, index (row) #3=2 ("disabled index (row)"), index (col) #3=w72, index (row) #4=3 ("disabled index (row)"), index (col) #4=w72, index (row) #5=4 ("disabled index (row)"), index (col) #5=w72, index (row) #6=5 ("index (col)"), index (col) #6=w72, index (row) #7=6 ("disabled index (row)"), index (col) #7=w72) -> (element #1=w103:string, element #2=w86:string, element #3=→"n meas":string, element #4=w81:string, element #5=w80:string, element #6=w78:string, element #7=w75:string)
            n23 = Decimal String To Number(string=w103) -> (number=w89:i32)  [unwired: 2 in, 1 out]
            n24 = Decimal String To Number(string=w81) -> (number=→"T wait start (s)":i32)  [unwired: 2 in, 1 out]
            n25 = Decimal String To Number(string=w80) -> (number=→"N meas stab":i32)  [unwired: 2 in, 1 out]
            n26 = Fract/Exp String To Number(string=w78) -> (number=→"Precisione mis":dbl)  [unwired: 3 in, 1 out]
            n27 = Fract/Exp String To Number(string=w75) -> (offset past number=→"T max misura":i32)  [unwired: 3 in, 1 out]
            n28 = Equal?(x=w86, y="1") -> (x = y?=w84:bool)
            n29 = local write "Mode sing?"(w84) -> ()
            n30 = Bundle By Name(cluster=T1 {"COM-Port (0)"=3, "Baud Rate (9600)"=9600, "Time-out (1.0)"=1.0, "Group Address (0)"=0, "Reset Device (Don't Reset)"=FALSE} ("Communication settings"), "COM-Port (0)"=w89) -> (w101:T1)
            "Communication settings" <- w101
            n31 = Unbundle By Name(w101) -> ("COM-Port (0)"=w97:i32, "Baud Rate (9600)"=w106:i32, "Time-out (1.0)"=w105:dbl, "Group Address (0)"=w104:i32, "Reset Device (Don't Reset)"=w71:bool)
            "COM-Port (0)" <- w97
            "Baud Rate (9600)" <- w106
            "Time-out (1.0)" <- w105
            "Group Address (0)" <- w104
            "Reset Device (Don't Reset)" <- w71
            n32 = call <instrlib>:"bp2316 Initialize.vi"("COM-Port (0)"=w97, "Baud Rate (9600)"=w106, "Time-out (1.0)"=w105, "error in (no error)"=w107, "Group Address (0)"=w104, "Reset Device (Don't Reset)"=w71) -> ("Instrument ID"=w96:i32, "error out"=w100:errorcluster)  [unwired: 7 in, 1 out]
            n33 = Equal To 0?(x=w96) -> (x = 0?=w99:bool)
            n34 = Bundle By Name(cluster=w100, "status"=w99) -> (w98:errorcluster)
          }
          frame True {
          }
        }
        n35 = flat-sequence {
          tunnel: w59 -> [w69]
          tunnel: w58 -> [_]
          frame #0 {
            n36 = Bundle By Name(cluster=cluster{"String":string, "variant":variant} {"String"="CONFIGURE", "variant"=variant} ("Single element"), "variant"=u16 2) -> (w66:cluster{"String":string, "variant":variant})
            n37 = Enqueue Element(queue=w69, element=w66) -> ()  [unwired: 2 in, 3 out]
          }
        }
        n38 = local write "MEASURE"(FALSE ("MEASURE")) -> ()
        n39 = control-ref of="This VI"() -> (w65:refnum<vi>)
        n40 = local write "stop"(FALSE ("stop")) -> ()
      }
      frame "CONFIGURE" {
        # "2mohm::SENS:FRES:RANG:MAN 2MOHM\n20mohm::SENS:FRES:RANG:MAN 20MOHM\n200ohm::SENS:FRES:RANG:MAN 200MOHM\n2ohm::SENS:FRES:RANG:MAN 2OHM\n20ohm::SENS:FRES:RANG:MAN 20OHM\n200ohm::SENS:FRES:RANG:MAN 200OHM\n2Kohm::SENS:FRES:RANG:MAN 2KOHM\n20Kohm::SENS:FRES:RANG:MAN 20KOHM\n200Kohm::SENS:FRES:RANG:MAN 200KOHM\n\nstatus query :: SENS:FRES:RANG:MAN?"
        n41 = Variant To Data(type=u16 0, Variant=w124) -> (data=w122:u16)  [unwired: 1 in, 1 out]
        "SCALA" <- w122
        n42 = local read "n meas"() -> (w118:string)
        n43 = Select(t="CALC:LIM:CONT:DATA " ("sendSCPIMessage"), s="Mode sing?", f="SENS:AVER:COUN" ("sendSCPIMessage")) -> (s? t:f=w110:string)
        n44 = Select(t="SENS:FRES:MODE SING " ("sendSCPIMessage"), s="Mode sing?", f="SENS:FRES:MODE CONT " ("sendSCPIMessage")) -> (s? t:f=w113:string)
        n45 = Index Array(array=string[] ["20MOHM", "200MOHM", "2OHM", "20OHM", "200OHM", "2KOHM", "20KOHM", "200KOHM"], index=w122) -> (element=w120:string)
        n46 = Concatenate Strings(w110, w118) -> (w117:string)
        n47 = Concatenate Strings("SENS:FRES:RANG:MAN " ("sendSCPIMessage"), w120) -> (w119:string)
        n48 = Build Array(w113, "SENS:FRES:RANG:AUTO 0" ("sendSCPIMessage"), w117, w119) -> (w126:string[])
        n49 = case shown="False" w116 {
          tunnel: w129 -> [w142 w147]
          tunnel: [w132 w147] -> w128
          tunnel: w126 -> [w141 _]
          frame False {
            w139 = "1" ("search string")
            n50 = for {
              shift-right: [w145] -> w136
              shift-left: w142 -> [w146]
              tunnel: w141 -> [w144] mode=indexing
              i -> [w143]
              n51 = call <instrlib>:"bp2316 Send A SCPI-Message.vi"("error in (no error)"=w146, "Send-SCPI-Message"=w144) -> ("error out"=w145:errorcluster)  [unwired: 8 in, 1 out]
              "Iteration" <- w143
            }
            n52 = call <instrlib>:"bp2316 Receive A SCPI-Message.vi"("error in (no error)"=w136, "Send-SCPI-Message"="*TST?") -> ("Instrument Answers"=w138:string)  [unwired: 7 in, 2 out]
            n53 = Search and Replace String(input string=w138, search string=w139, replace string=w139) -> (number of replacements=w140:i32)  [unwired: 5 in, 3 out]
            n54 = Greater Than 0?(x=w140) -> (x > 0?=w133:bool)
            n55 = Select(t=errorcluster {"status"=FALSE, "code"=0, "source"=""} ("error out"), s=w133, f=errorcluster {"status"=TRUE, "code"=0, "source"=""} ("error out")) -> (s? t:f=w132:errorcluster)
          }
          frame True {
          }
        }
      }
      frame "START RES" {
        (unwired) TRUE  # AVV. avviamento?
        n56 = case shown="False" w155 {
          tunnel: w148 -> [w157 w190]
          tunnel: [w158 w190] -> w151
          frame False {
            n57 = while {
              shift-right: [w166] -> w158
              shift-left: w157 -> [_]
              i -> [w179]
              stop <- w180 stop-if-true
              w170 = "1" ("search string")
              n58 = local read "COM-Port (0)"() -> (w162:i32)
              n59 = call <instrlib>:"bp2316 Initialize.vi"("COM-Port (0)"=w162) -> ("Instrument ID"=w161:i32, "error out"=w176:errorcluster)  [unwired: 12 in, 1 out]
              n60 = Equal To 0?(x=w161) -> (x = 0?=w174:bool)
              n61 = Or(x=w174, y=w176) -> (x .or. y?=w175:bool)
              n62 = case shown="False" w175 {
                tunnel: w161 -> [w183 w186]
                tunnel: [w182 w184] -> w167
                tunnel: [w183 w185] -> w173
                tunnel: w176 -> [w182 _]
                frame False {
                }
                frame True {
                  n63 = flat-sequence {
                    tunnel: w186 -> [w187]
                    tunnel: [w188] -> w185
                    tunnel: [w189] -> w184
                    frame #0 {
                      n64 = call <instrlib>:"bp2316 Close.vi"("Instrument ID (1)"=w187) -> ()  [unwired: 9 in, 2 out]
                    }
                    frame #1 {
                      n65 = call <instrlib>:"bp2316 Initialize.vi"() -> ("Instrument ID"=w188:i32, "error out"=w189:errorcluster)  [unwired: 13 in, 1 out]
                    }
                  }
                }
              }
              n66 = Equal To 0?(x=w173) -> (x = 0?=w172:bool)
              n67 = call <instrlib>:"bp2316 Receive A SCPI-Message.vi"("error in (no error)"=w167, "Send-SCPI-Message"="*TST?") -> ("error out"=w166:errorcluster, "Instrument Answers"=w169:string)  [unwired: 7 in, 1 out]
              n68 = Search and Replace String(input string=w169, search string=w170, replace string=w170) -> (number of replacements=w171:i32)  [unwired: 5 in, 3 out]
              n69 = Greater Than 0?(x=w171) -> (x > 0?=w163:bool)
              n70 = Not(x=w172) -> (.not. x?=w181:bool)
              n71 = Select(t=errorcluster {"status"=FALSE, "code"=0, "source"=""} ("error out"), s=w163, f=errorcluster {"status"=TRUE, "code"=0, "source"=""} ("error out")) -> (s? t:f=w159:errorcluster)
              n72 = Greater?(x=w179, y=1) -> (0:w177:bool)
              n73 = Or(x=w181, y=w177) -> (x .or. y?=w180:bool)
              n74 = call "SEND STATUS.vi"("ELEMENT"=DEVICE_NAME."RESISTOMAT", "error in (no error)"=w159) -> ()  [unwired: 9 in, 1 out]
            }
          }
          frame True {
          }
        }
        n75 = Enqueue Element(queue=w150, element=cluster{"String":string, "variant":variant} {"String"="READ", "variant"=variant} ("Single element")) -> ()  [unwired: 2 in, 3 out]
        n76 = local write "MEASURE"(TRUE ("MEASURE")) -> ()
        n77 = Unbundle By Name(w151) -> ("status"=w154:bool)
        n78 = Not(x=w154) -> (.not. x?=w153:bool)
      }
      frame "STOP RES" {
        n79 = case shown="False" w192 {
          tunnel: w194 -> [w197 w198]
          tunnel: [w196 w198] -> w193
          frame False {
            n80 = call <instrlib>:"bp2316 Measure Stop.vi"("error in (no error)"=w197) -> ("error out"=w196:errorcluster)  [unwired: 9 in, 1 out]
          }
          frame True {
          }
        }
        n81 = local write "MEASURE"(FALSE ("MEASURE")) -> ()
      }
      frame "READ" {
        n82 = case shown="False" w210 {
          tunnel: w216 -> [w229 w254]
          tunnel: [w229 w254] -> w208
          tunnel: [w233 w249] -> w199
          tunnel: w215 -> [_ w252]
          tunnel: [w234 w246] -> _
          tunnel: [w232 _] -> w214
          tunnel: [w231 1 ("instrument ID")] -> w211
          frame False {
            w231 = 1 ("instrument ID")
            n83 = local read "SCALA"() -> (w223:u16)
            n84 = local read "Precisione mis"() -> (w225:dbl)
            n85 = local read "T wait start (s)"() -> (w224:i32)
            n86 = local read "T max misura"() -> (w228:i32)
            n87 = local read "N meas stab"() -> (w226:i32)
            n88 = local read "COM-Port (0)"() -> (w230:i32)
            n89 = local read "Mode sing?"() -> (w227:bool)
            n90 = call "Resistomat_2316_2.vi"("Scala resistomat"=w223, "instrument ID"=w231, "N meas stab"=w226, "Precisione"=w225, "T after start"=w224, "Time bef err"=w228, "COM-Port (0)"=w230, "Sing?"=w227) -> ("seconds since 1Jan1904"=w234:timestamp, "Measuring Value (ohm)"=w233:dbl, "errore resistomat"=w232:bool)  [unwired: 16 in, 1 out]
            "errore resistomat" <- w232
          }
          frame True {
            (unwired) "SIMULAZIONE" ("Unit")
            n91 = global read "Global_All_Data.vi" "All Data"() -> (w242:T3)
            n92 = Unbundle By Name(w242) -> ("MISURE NM.t. acq [min]"=w241:string)
            n93 = Fract/Exp String To Number(string=w241) -> (number=w240:dbl)  [unwired: 3 in, 1 out]
            n94 = Divide(x=w240, y=2.0) -> (x/y=w243:dbl)
            n95 = Hyperbolic Tangent(1:w243) -> (0:w239:dbl)
            n96 = Divide(x=w239, y=4.0) -> (x/y=w235:dbl)
            n97 = Add(x=w235, y=3.25) -> (x+y=w237:dbl)
            n98 = Wait (ms)(milliseconds to wait=u32 400) -> ()  [unwired: 1 out]
            n99 = call <userlib>:"MEASURE SIMULATOR.vi"("delay (100)"=u32 1, "precision %"=0.1, "amplitude"=w237) -> ("value"=w251:dbl)  [unwired: 8 in]
            n100 = Get Date/Time In Seconds() -> (seconds since 1Jan1904=w246:timestamp)
            n101 = Select(t=w251, s=w252, f=0.0) -> (s? t:f=w249:dbl)
          }
        }
        "Measuring Value" <- w199
        n102 = case shown="False" w210 {
          tunnel: w211 -> [w220 w222]
          tunnel: w208 -> [w221 _]
          tunnel: [w220 w222] -> w204
          frame False {
            n103 = call <instrlib>:"bp2316 Measure Stop.vi"("error in (no error)"=w221, "Instrument ID (1)"=w220) -> ()  [unwired: 8 in, 2 out]
          }
          frame True {
          }
        }
        n104 = Equal?(x=w199, y=-1.0) -> (x = y?=w212:bool)
        n105 = Or(x=w212, y=w214) -> (x .or. y?=w209:bool)
        n106 = Obtain Notifier(name (unnamed)="Misura resistomat", notification data type=0.0 ("misura res")) -> (notifier out=w202:refnum<notifier>, error out=w203:errorcluster)  [unwired: 2 in, 1 out]
        n107 = Send Notification(notification=w199, notifier=w202, error in (no error)=w203) -> ()  [unwired: 2 out]
        n108 = case shown="True" w209 {
          tunnel: w204 -> [_ w218]
          frame False {
          }
          frame True {
            n109 = global read "Stop lettura res.vi" "STOP LETTURA RES"() -> (w219:bool)
            n110 = call <instrlib>:"bp2316 Measure Stop.vi"("Instrument ID (1)"=w218) -> ()  [unwired: 9 in, 2 out]
            n111 = case shown="True" w219 {
              frame False {
                # "mettere \navviso\nerrore\nres"
              }
              frame True {
              }
            }
          }
        }
        n112 = Bundle By Name(cluster=cluster{"String":string, "variant":variant} {"String"="Acquisisci misura res", "variant"=variant} ("element"), "variant"=w199) -> (w205:cluster{"String":string, "variant":variant})
        n113 = Enqueue Element(queue=w207, element=w205) -> ()  [unwired: 2 in, 3 out]
      }
      frame "CALCOLA RES0" {
        # "T2=(R2/R1)*(235+T1)-235"
      }
      frame "OPEN" {
        n114 = call <userlib>:"easy open VI panel.vi"("VI in"=w258) -> ()  [unwired: 10 in, 1 out]
      }
      frame "STOP RESISTENZE" {
        n115 = Flush Queue(queue=w264, error in (no error)=w263) -> (error out=w262:errorcluster)  [unwired: 2 out]
        n116 = call <instrlib>:"bp2316 Measure Stop.vi"("error in (no error)"=w262, "Instrument ID (1)"=1) -> ("error out"=w261:errorcluster)  [unwired: 8 in, 1 out]
      }
      frame "Exit" {
        n117 = property on="stop" class="Bool (strict)"("Val(Sgnl)"=TRUE ("Value (Signaling)")) -> ()  [unwired: 2 in, 2 out]
        n118 = case shown="False" w269 {
          tunnel: w268 -> [w273 w274]
          tunnel: [w272 w274] -> w267
          frame False {
            n119 = call <instrlib>:"bp2316 Close.vi"("error in (no error)"=w273) -> ("error out"=w272:errorcluster)  [unwired: 9 in, 1 out]
          }
          frame True {
          }
        }
      }
    }
    n120 = Or(x=FALSE, y=w46) -> (x .or. y?=w35:bool)
    n121 = call "SEND STATUS.vi"("ELEMENT"=DEVICE_NAME."RESISTOMAT", "error in (no error)"=w30) -> ()  [unwired: 9 in, 1 out]
    "Numeric" <- w29
  }
  n122 = while {
    tunnel: w7 -> [w275]
    stop <- w276 stop-if-true
    # "PROCESSI A EVENTI"
    n123 = event shown="[3] \"stop\": Value Change" {
      selector: _ -> [_ _ _ _]
      dyn-events: _ -> [_ _ _ _]
      timeout: _ -> [_ _ _ _]
      tunnel: [_ _ _ w295] -> w276
      tunnel: w275 -> [w282 _ w289 _]
      event "MEASURE": Value Change {
        n124 = event-data() -> ("NewVal"=w283:bool)  [unwired: 1 in]
        n125 = local read "RANGE"() -> (w278:u16)
        n126 = Bundle By Name(cluster=cluster{"String":string, "variant":variant} {"String"="START RES", "variant"=variant} ("Single element"), "variant"=w278) -> (w279:cluster{"String":string, "variant":variant})
        n127 = Select(t=w279, s=w283, f=cluster{"String":string, "variant":variant} {"String"="STOP RES", "variant"=variant} ("Single element")) -> (s? t:f=w281:cluster{"String":string, "variant":variant})
        n128 = Enqueue Element(queue=w282, element=w281) -> ()  [unwired: 2 in, 3 out]
      }
      event "Misura Resistomat": Value Change {
        n129 = event-data() -> ()  [unwired: 1 in, 6 out]
        n130 = Obtain Notifier(name (unnamed)="Misura resistomat", notification data type=0.0 ("misura res")) -> (notifier out=w286:refnum<notifier>, error out=w285:errorcluster)  [unwired: 2 in, 1 out]
        n131 = Send Notification(notification=1.22, notifier=w286, error in (no error)=w285) -> ()  [unwired: 2 out]
      }
      event "CONFIGURE": Value Change {
        n132 = event-data() -> ("NewVal"=w290:bool)  [unwired: 1 in]
        n133 = case shown="True" w290 {
          tunnel: w289 -> [_ w293]
          frame False {
          }
          frame True {
            n134 = Bundle By Name(cluster=cluster{"String":string, "variant":variant} {"String"="CONFIGURE", "variant"=variant} ("Single element"), "variant"="RANGE") -> (w291:cluster{"String":string, "variant":variant})
            n135 = Enqueue Element(queue=w293, element=w291) -> ()  [unwired: 2 in, 3 out]
          }
        }
      }
      event "stop": Value Change {
        n136 = event-data() -> ("NewVal"=w295:bool)  [unwired: 1 in, 5 out]
      }
    }
  }
  n137 = property on="stop" class="Bool (strict)"("Val(Sgnl)"=w15) -> ()  [unwired: 2 in, 2 out]
  n138 = flat-sequence {
    tunnel: w18 -> [w301]
    tunnel: w4 -> [w296]
    frame #0 {
      n139 = property class="VI"(reference=w301) -> (reference out=w297:refnum<vi>, "FP.State"=w300:T30)  [unwired: 1 in, 1 out]
      n140 = Not Equal?(x=T30."Closed", y=w300) -> (x != y?=w298:bool)
      n141 = case shown="True" w298 {
        tunnel: w297 -> [_ w302]
        frame False {
        }
        frame True {
          n142 = invoke class="VI" method="FP.Close"(reference=w302) -> ()  [unwired: 2 in, 3 out]
        }
      }
      "error out" <- w296
    }
  }
